vi "Tree_UsbScShdlc_Sensirion.vi"   [LabVIEW 2012]
doc: "Tree_UsbScShdlc_Sensirion.vi\n----------------------------------------------\n\nThis is the tree VI for USB Sensor Cable commands.\n\n----------------------------------------------\n24.09.2015, Thomas Huber\n\nSensirion AG\nCH-8712 Stäfa ZH\nwww.sensirion.com"
panel:
  # "SEE DIAGRAM\nFOR VI TREE."
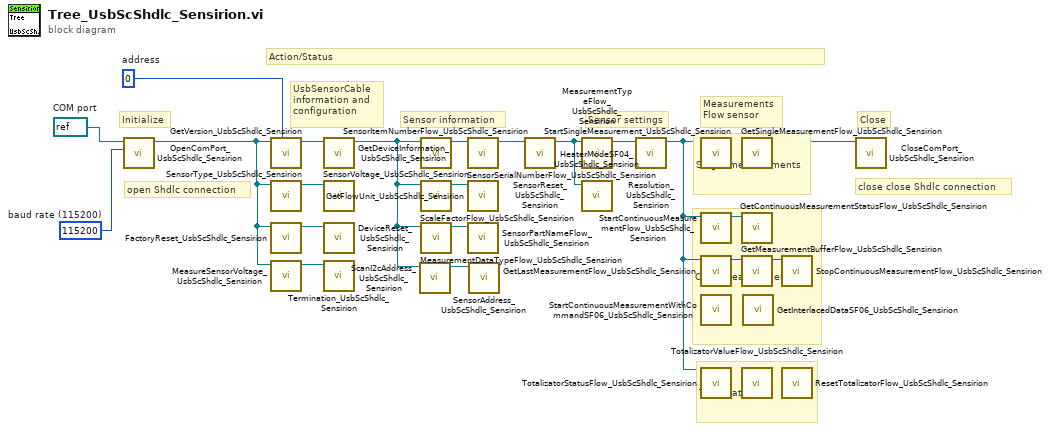
[diagram p0: block diagram]
diagram:
  w21 = u32 115200  # baud rate (115200)
  w22 = refnum<visa-resource-name> refnum  # COM port
  w23 = u8 0  # address
  # "Measurements\nFlow sensor"
  # "Sensor settings"
  # "Sensor information"
  # "UsbSensorCable \ninformation and \nconfiguration"
  # "close close Shdlc connection"
  # "open Shdlc connection"
  # "Action/Status"
  # "Close"
  # "Initialize"
  # "Cont. measurements"
  # "Totalizator"
  # "Single measurements"
  n1 = call "OpenComPort_UsbScShdlc_Sensirion.vi"("baud rate (115200)"=w21, "COM port"=w22) -> ("COM port out"=w18:refnum<visa-resource-name>)  [unwired: 8 in, 1 out]
  n2 = call "GetVersion_UsbScShdlc_Sensirion.vi"("address"=w23, "COM port"=w18) -> ("COM port out"=w24:refnum<visa-resource-name>)  [unwired: 7 in, 2 out]
  n3 = call "SensorType_UsbScShdlc_Sensirion.vi"("COM port"=w18) -> ("COM port out"=w20:refnum<visa-resource-name>)  [unwired: 8 in, 2 out]
  n4 = call "FactoryReset_UsbScShdlc_Sensirion.vi"("COM port"=w18) -> ("COM port out"=w19:refnum<visa-resource-name>)  [unwired: 9 in, 1 out]
  n5 = call "MeasureSensorVoltage_UsbScShdlc_Sensirion.vi"("COM port"=w18) -> ("COM port out"=w17:refnum<visa-resource-name>)  [unwired: 8 in, 2 out]
  n6 = call "GetDeviceInformation_UsbScShdlc_Sensirion.vi"("COM port"=w24) -> ("COM port out"=w3:refnum<visa-resource-name>)  [unwired: 8 in, 2 out]
  n7 = call "SensorVoltage_UsbScShdlc_Sensirion.vi"("COM port"=w20) -> ()  [unwired: 8 in, 3 out]
  n8 = call "DeviceReset_UsbScShdlc_Sensirion.vi"("COM port"=w19) -> ()  [unwired: 9 in, 2 out]
  n9 = call "Termination_UsbScShdlc_Sensirion.vi"("COM port"=w17) -> ()  [unwired: 8 in, 3 out]
  n10 = call "ScanI2cAddress_UsbScShdlc_Sensirion.vi"("COM port"=w3) -> ("COM port out"=w2:refnum<visa-resource-name>)  [unwired: 8 in, 2 out]
  n11 = call "SensorItemNumberFlow_UsbScShdlc_Sensirion.vi"("COM port"=w3) -> ("COM port out"=w16:refnum<visa-resource-name>)  [unwired: 8 in, 2 out]
  n12 = call "ScaleFactorFlow_UsbScShdlc_Sensirion.vi"("COM port"=w3) -> ("COM port out"=w15:refnum<visa-resource-name>)  [unwired: 8 in, 2 out]
  n13 = call "MeasurementDataTypeFlow_UsbScShdlc_Sensirion.vi"("COM port"=w3) -> ("COM port out"=w1:refnum<visa-resource-name>)  [unwired: 8 in, 2 out]
  n14 = call "SensorSerialNumberFlow_UsbScShdlc_Sensirion.vi"("COM port"=w16) -> ("COM port out"=w14:refnum<visa-resource-name>)  [unwired: 8 in, 2 out]
  n15 = call "GetFlowUnit_UsbScShdlc_Sensirion.vi"("COM port"=w15) -> ()  [unwired: 8 in, 3 out]
  n16 = call "SensorPartNameFlow_UsbScShdlc_Sensirion.vi"("COM port"=w1) -> ()  [unwired: 8 in, 3 out]
  n17 = call "SensorAddress_UsbScShdlc_Sensirion.vi"("COM port"=w2) -> ()  [unwired: 8 in, 3 out]
  n18 = call "SensorReset_UsbScShdlc_Sensirion.vi"("COM port"=w14) -> ("COM port out"=w12:refnum<visa-resource-name>)  [unwired: 9 in, 1 out]
  n19 = call "MeasurementTypeFlow_UsbScShdlc_Sensirion.vi"("COM port"=w12) -> ("COM port out"=w13:refnum<visa-resource-name>)  [unwired: 8 in, 2 out]
  n20 = call "HeaterModeSF04_UsbScShdlc_Sensirion.vi"("COM port"=w12) -> ()  [unwired: 8 in, 3 out]
  n21 = call "Resolution_UsbScShdlc_Sensirion.vi"("COM port"=w13) -> ("COM port out"=w7:refnum<visa-resource-name>)  [unwired: 8 in, 2 out]
  n22 = call "StartSingleMeasurement_UsbScShdlc_Sensirion.vi"("COM port"=w7) -> ("COM port out"=w11:refnum<visa-resource-name>)  [unwired: 9 in, 1 out]
  n23 = call "StartContinuousMeasurementFlow_UsbScShdlc_Sensirion.vi"("COM port"=w7) -> ("COM port out"=w10:refnum<visa-resource-name>)  [unwired: 9 in, 1 out]
  n24 = call "GetLastMeasurementFlow_UsbScShdlc_Sensirion.vi"("COM port"=w7) -> ("COM port out"=w9:refnum<visa-resource-name>)  [unwired: 7 in, 3 out]
  n25 = call "StartContinuousMeasurementWithCommandSF06_UsbScShdlc_Sensirion.vi"() -> ()  [unwired: 10 in, 2 out]
  n26 = call "TotalizatorStatusFlow_UsbScShdlc_Sensirion.vi"("COM port"=w7) -> ("COM port out"=w6:refnum<visa-resource-name>)  [unwired: 8 in, 2 out]
  n27 = call "GetSingleMeasurementFlow_UsbScShdlc_Sensirion.vi"("COM port"=w11) -> ("COM port out"=w4:refnum<visa-resource-name>)  [unwired: 7 in, 3 out]
  n28 = call "GetContinuousMeasurementStatusFlow_UsbScShdlc_Sensirion.vi"("COM port"=w10) -> ()  [unwired: 8 in, 3 out]
  n29 = call "GetMeasurementBufferFlow_UsbScShdlc_Sensirion.vi"("COM port"=w9) -> ("COM port out"=w8:refnum<visa-resource-name>)  [unwired: 6 in, 4 out]
  n30 = call "TotalizatorValueFlow_UsbScShdlc_Sensirion.vi"("COM port"=w6) -> ("COM port out"=w5:refnum<visa-resource-name>)  [unwired: 8 in, 2 out]
  n31 = call "GetInterlacedDataSF06_UsbScShdlc_Sensirion.vi"() -> ()  [unwired: 8 in, 4 out]
  n32 = call "StopContinuousMeasurementFlow_UsbScShdlc_Sensirion.vi"("COM port"=w8) -> ()  [unwired: 9 in, 2 out]
  n33 = call "ResetTotalizatorFlow_UsbScShdlc_Sensirion.vi"("COM port"=w5) -> ()  [unwired: 9 in, 2 out]
  n34 = call "CloseComPort_UsbScShdlc_Sensirion.vi"("COM port"=w4) -> ()  [unwired: 10 in, 1 out]
